vi "Control, Center X.vi"(0 "error in":errorcluster, 3 "Ctl ref":refnum<vi>, 4 "X (0)":i32) -> (7 "error out":errorcluster, 10 "Ctl ref dup":refnum<vi>)   [LabVIEW 2010]
doc: "This function centers a GUI control on a vertical axis."
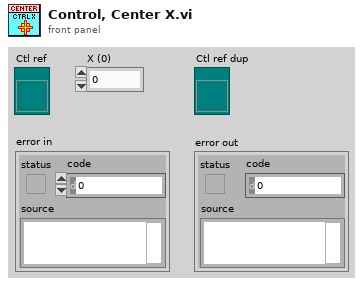
[diagram p1: front panel]
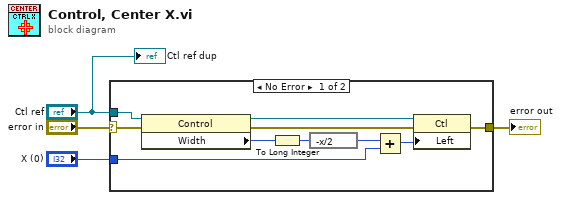
[diagram p0: block diagram]
diagram:
  n1 = case shown="No Error" "error in" {
    selector: "error in" -> [w13 w15]
    tunnel: [w11 w15] -> w4
    tunnel: "Ctl ref" -> [w14 _]
    tunnel: "X (0)" -> [w9 _]
    frame No Error {
      n2 = property class="Control"(reference=w14, error in=w13) -> (reference out=w5:refnum<vi>, error out=w12:errorcluster, "Width"=w8:u32)
      n3 = To Long Integer(number=w8) -> (32bit integer=w7:i32)
      n4 = expression code="-x/2"(w7) -> (w6:i32)
      n5 = Add(x=w6, y=w9) -> (x+y=w10:i32)
      n6 = property class="Ctl"(reference=w5, error in=w12, "Left"=w10) -> (error out=w11:errorcluster)  [unwired: 1 out]
    }
    frame Error {
    }
  }
  "error out" <- w4
  "Ctl ref dup" <- "Ctl ref"
